vi "fpga_16ch-SchedulerOV.vi"() -> (0 "overflow":bool, 1 "FIFO Schedule":u8, 2 "Main clock":u32)   [LabVIEW 2011]
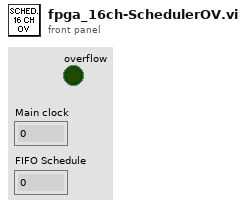
[diagram p1: front panel]
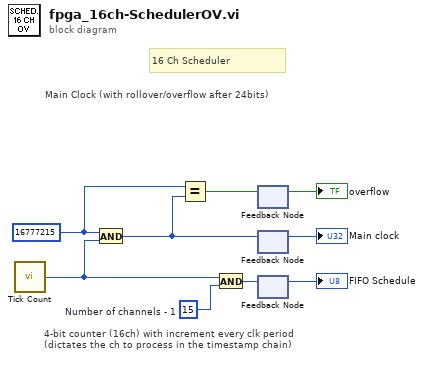
[diagram p0: block diagram]
diagram:
  w1 = u32 16777215 ("x")
  w9 = u32 15  # Number of channels - 1
  # "16 Ch Scheduler"
  # "Main Clock (with rollover/overflow after 24bits)"
  # "4-bit counter (16ch) with increment every clk period\n(dictates the ch to process in the timestamp chain)"
  n1 = call "Tick Count"() -> ("Tick Count(Ticks)"=w5:u32)
  n2 = And(x=w1, y=w5) -> (x .and. y?=w4:u32)
  n3 = Equal?(x=w1, y=w4) -> (x = y?=w2:bool)
  n4 = And(x=w5, y=w9) -> (x .and. y?=w8:u32)
  n5 = feedback #1() -> (→"overflow":bool)  [unwired: 1 in]
  n6 = feedback-in #1(w2) -> ()
  n7 = feedback-in #2(w4) -> ()
  n8 = feedback #2() -> (→"Main clock":u32)  [unwired: 1 in]
  n9 = feedback-in #3(w8) -> ()
  n10 = feedback #3() -> (→"FIFO Schedule":u32)  [unwired: 1 in]
